vi "Y Axis Motor state control subVI.vi"(8 "error in (no error)":errorcluster, 10 "stop":bool, 11 "Y Axis Motor Target":T1) -> (0 "error out":errorcluster, 3 "Y Axis Motor Params":T1)   [LabVIEW 2017]
uses:
  Motor Status Enum.ctl
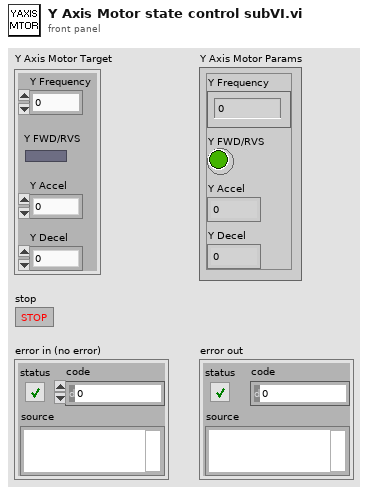
[diagram p1: front panel]
types:
  T1 = cluster{"Y Frequency":dbl, "Y FWD/RVS":bool, "Y Accel":dbl, "Y Decel":dbl}
  T2 = cluster{"Y Frequency":dbl, "Y FWD/RVS":bool, "Accel":dbl, "Decel":dbl}
  T3 = typedef "Motor Status Enum.ctl" = enum16{"Stop Motor", "Read Inputs", "Steady Speed", "Accelerate", "Decelerate"}
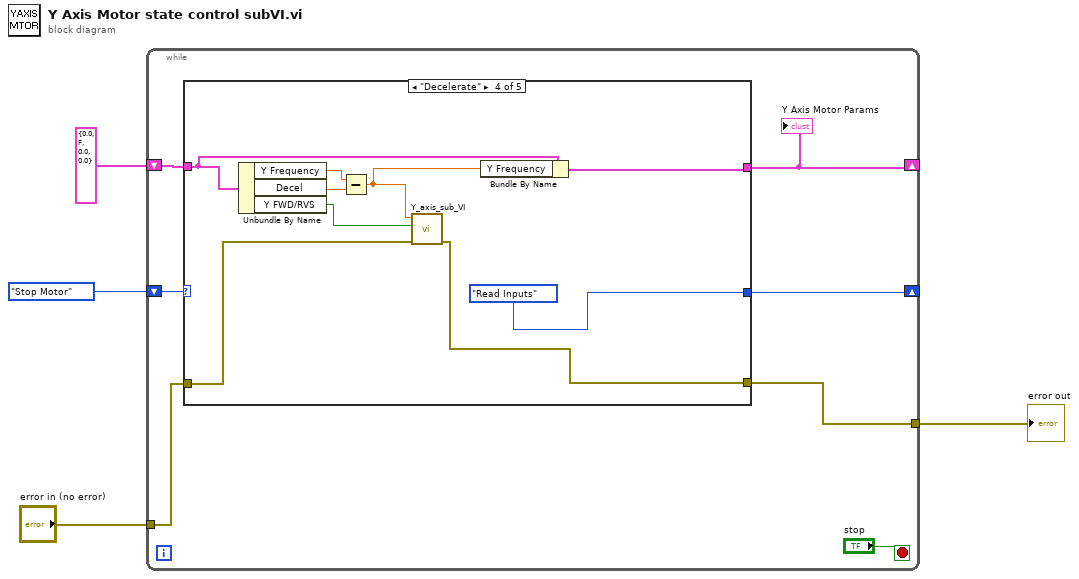
[diagram p0: block diagram]
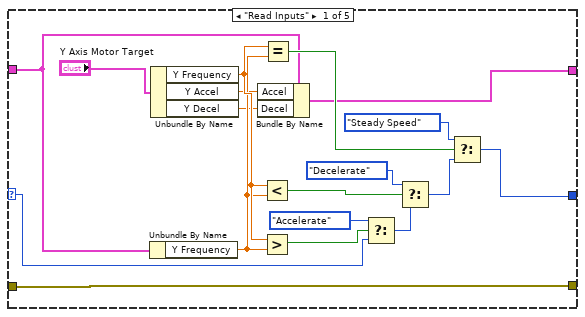
[diagram p2: hidden frame]
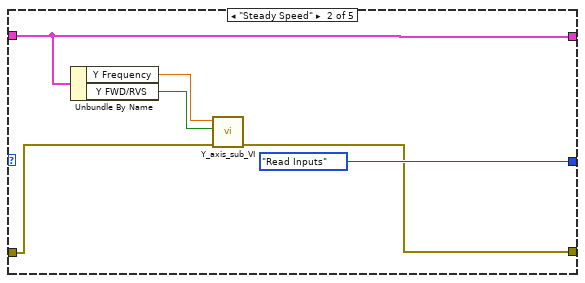
[diagram p3: hidden frame]
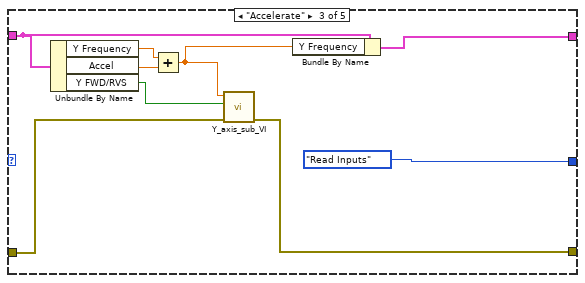
[diagram p4: hidden frame]
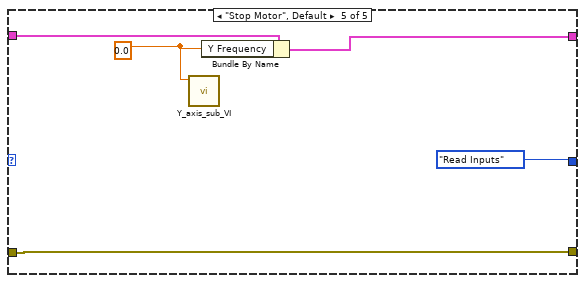
[diagram p5: hidden frame]
diagram:
  n1 = while {
    shift-right: [w10] -> _
    shift-left: Motor_Status_Enum."Stop Motor" -> [w11]
    shift-right: [w8] -> _
    shift-left: T2 {"Y Frequency"=0.0, "Y FWD/RVS"=FALSE, "Accel"=0.0, "Decel"=0.0} ("Y Axis Motor Params 2") -> [w9]
    tunnel: "error in (no error)" -> [w7]
    tunnel: [w6] -> w3
    stop <- "stop" stop-if-true
    n2 = case shown="\"Decelerate\"" w11 {
      selector: w11 -> [w26 _ _ _ _]
      tunnel: [w17 Motor_Status_Enum."Read Inputs" Motor_Status_Enum."Read Inputs" Motor_Status_Enum."Read Inputs" Motor_Status_Enum."Read Inputs"] -> w10
      tunnel: [w15 w30 w40 w50 w57] -> w8
      tunnel: w9 -> [w14 w30 w44 w49 w56]
      tunnel: w7 -> [w16 w34 w42 w48 w54]
      tunnel: [w16 w33 w41 w47 w54] -> w6
      frame "Read Inputs" {
        n3 = Unbundle By Name(w14) -> ("Y Frequency"=w21:dbl)
        n4 = Unbundle By Name("Y Axis Motor Target") -> ("Y Frequency"=w22:dbl, "Y Accel"=w13:dbl, "Y Decel"=w12:dbl)
        n5 = Bundle By Name(cluster=w14, "Accel"=w13, "Decel"=w12) -> (w15:T2)
        n6 = Less?(x=w22, y=w21) -> (x < y?=w25:bool)
        n7 = Greater?(x=w22, y=w21) -> (0:w28:bool)
        n8 = Equal?(x=w22, y=w21) -> (x = y?=w20:bool)
        n9 = Select(t=Motor_Status_Enum."Accelerate", s=w28, f=w26) -> (s? t:f=w23:T3)
        n10 = Select(t=Motor_Status_Enum."Decelerate", s=w25, f=w23) -> (s? t:f=w19:T3)
        n11 = Select(t=Motor_Status_Enum."Steady Speed", s=w20, f=w19) -> (s? t:f=w17:T3)
      }
      frame "Steady Speed" {
        n12 = Unbundle By Name(w30) -> ("Y Frequency"=w32:dbl, "Y FWD/RVS"=w31:bool)
        n13 = call "Y_axis_sub_VI.vi"("error in (no error)"=w34, "FWD/RVS"=w31, "Frequency"=w32) -> ("error out"=w33:errorcluster)  [unwired: 8 in]
      }
      frame "Accelerate" {
        n14 = Unbundle By Name(w44) -> ("Y Frequency"=w39:dbl, "Accel"=w37:dbl, "Y FWD/RVS"=w36:bool)
        n15 = Add(x=w39, y=w37) -> (x+y=w38:dbl)
        n16 = call "Y_axis_sub_VI.vi"("error in (no error)"=w42, "FWD/RVS"=w36, "Frequency"=w38) -> ("error out"=w41:errorcluster)  [unwired: 8 in]
        n17 = Bundle By Name(cluster=w44, "Y Frequency"=w38) -> (w40:T2)
      }
      frame "Decelerate" {
        n18 = Unbundle By Name(w49) -> ("Y Frequency"=w51:dbl, "Decel"=w53:dbl, "Y FWD/RVS"=w45:bool)
        n19 = Subtract(x=w51, y=w53) -> (x-y=w52:dbl)
        n20 = call "Y_axis_sub_VI.vi"("error in (no error)"=w48, "FWD/RVS"=w45, "Frequency"=w52) -> ("error out"=w47:errorcluster)  [unwired: 8 in]
        n21 = Bundle By Name(cluster=w49, "Y Frequency"=w52) -> (w50:T2)
      }
      frame "Stop Motor", Default {
        w55 = 0.0 ("Y Frequency")
        n22 = call "Y_axis_sub_VI.vi"("Frequency"=w55) -> ()  [unwired: 10 in, 1 out]
        n23 = Bundle By Name(cluster=w56, "Y Frequency"=w55) -> (w57:T2)
      }
    }
    "Y Axis Motor Params" <- w8
  }
  "error out" <- w3
